vi "lab1.vi"() -> ()   [LabVIEW 2021]
panel:
  out "Напряжение":dbl(knob) scale=0.0..10.0
  out "Перегрузка":bool
  out "?":bool
  in  "Питание":bool
  in  "Порог":dbl(slide) scale=0.0..10.0
  in  "Напряжение":dbl(slide) scale=0.0..10.0
  in  "Шум":dbl(slide) scale=0.0..10.0
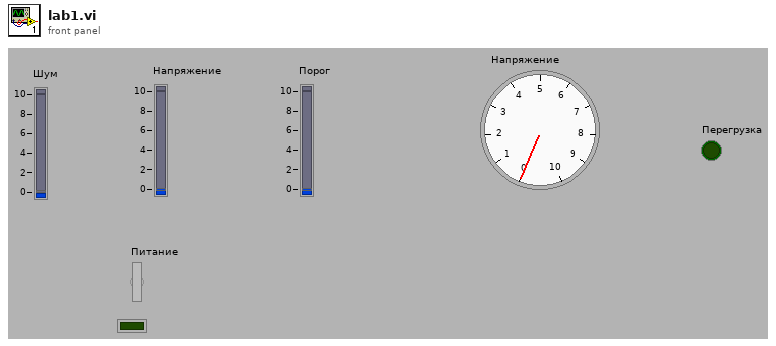
[diagram p1: front panel]
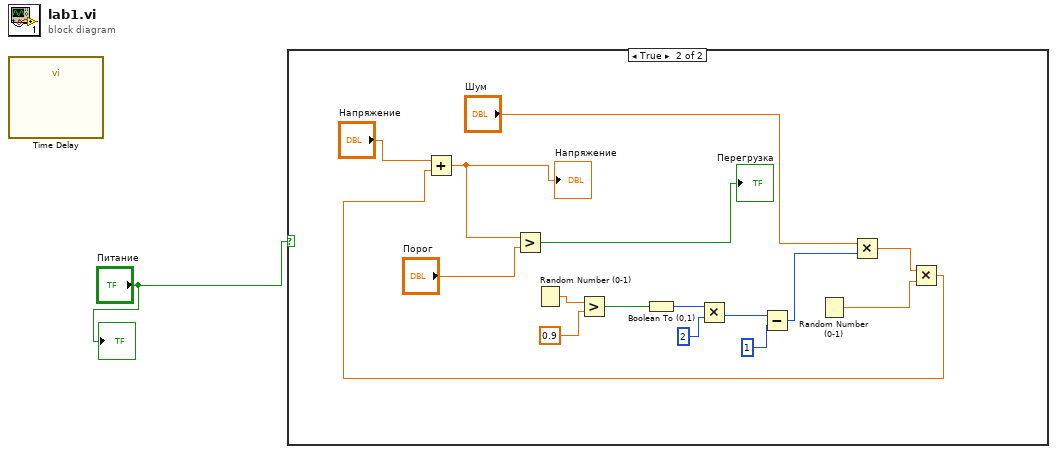
[diagram p0: block diagram]
diagram:
  n1 = call "Time Delay"() -> ()  [unwired: 11 in, 1 out]
  n2 = case shown="True" "Питание" {
    frame False {
    }
    frame True {
      n3 = Random Number (0-1)() -> (number: 0 to 1=w9:dbl)
      n4 = Greater?(x=w9, y=0.9) -> (0:w7:bool)
      n5 = Boolean To (0,1)(Boolean=w7) -> (0, 1=w6:i16)
      n6 = Multiply(x=w6, y=2) -> (x*y=w4:i32)
      n7 = Subtract(x=w4, y=1) -> (x-y=w2:i32)
      n8 = Random Number (0-1)() -> (number: 0 to 1=w11:dbl)
      n9 = Multiply(x="Шум", y=w2) -> (x*y=w12:dbl)
      n10 = Multiply(x=w12, y=w11) -> (x*y=w10:dbl)
      n11 = Add(x="Напряжение", y=w10) -> (x+y=w15:dbl)
      "Напряжение" <- w15
      n12 = Greater?(x=w15, y="Порог") -> (0:→"Перегрузка":bool)
    }
  }
  "?" <- "Питание"
